vi "CPP_ExponentialDecayFitDevelopment.vi"(4 "MedianFilter(points)":i32=3, 5 "SamplingRate":dbl, 6 "DecayData":dbl[](array[numeric]), 7 "FID ID":string) -> (0 "PlugInValues":string[](array[string]), 1 "smoothedCluster":T2, 2 "GraphClusterArray":T1(array[cluster]), 3 "PlugInTitles":string[](array[string]))   [LabVIEW 2012]
uses:
  <vilib>/measure/mascope.llb/Amplitude and Levels 1 chan.vi
  <vilib>/addons/Time Series Analysis/Series Preprocess.llb/TSA Moving Average (Array).vi
  <vilib>/Analysis/baseanly.llb/Mean (DBL).vi
  <vilib>/Analysis/NI_AALPro.lvlib
  <vilib>/Analysis/NI_AALBase.lvlib
  <vilib>/addons/_Advanced Signal Processing/NI_AdvSigProcTSA.lvlib
  <vilib>/measure/NI_MAPro.lvlib
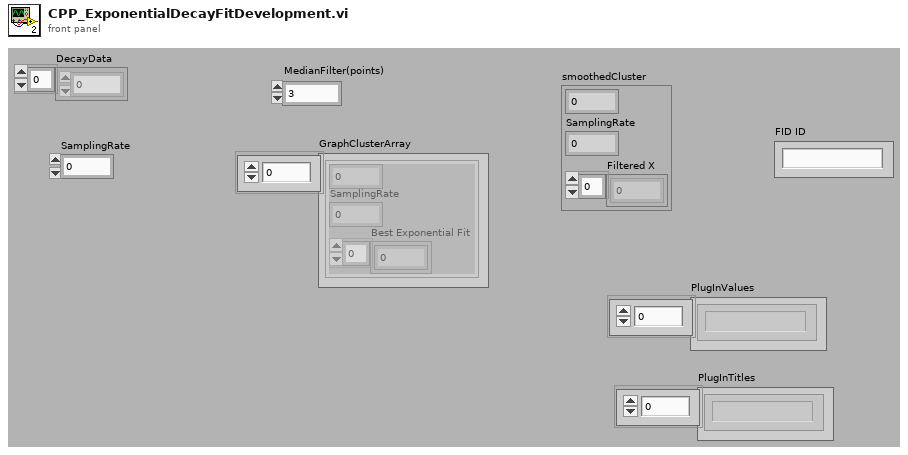
[diagram p1: front panel]
types:
  T1 = cluster{dbl, "SamplingRate":dbl, "Best Exponential Fit":dbl[]}[]
  T2 = cluster{"x*y":dbl, "SamplingRate":dbl, "Filtered X":dbl[]}
  T3 = cluster{dbl, "SamplingRate":dbl, "Best Exponential Fit":dbl[]}
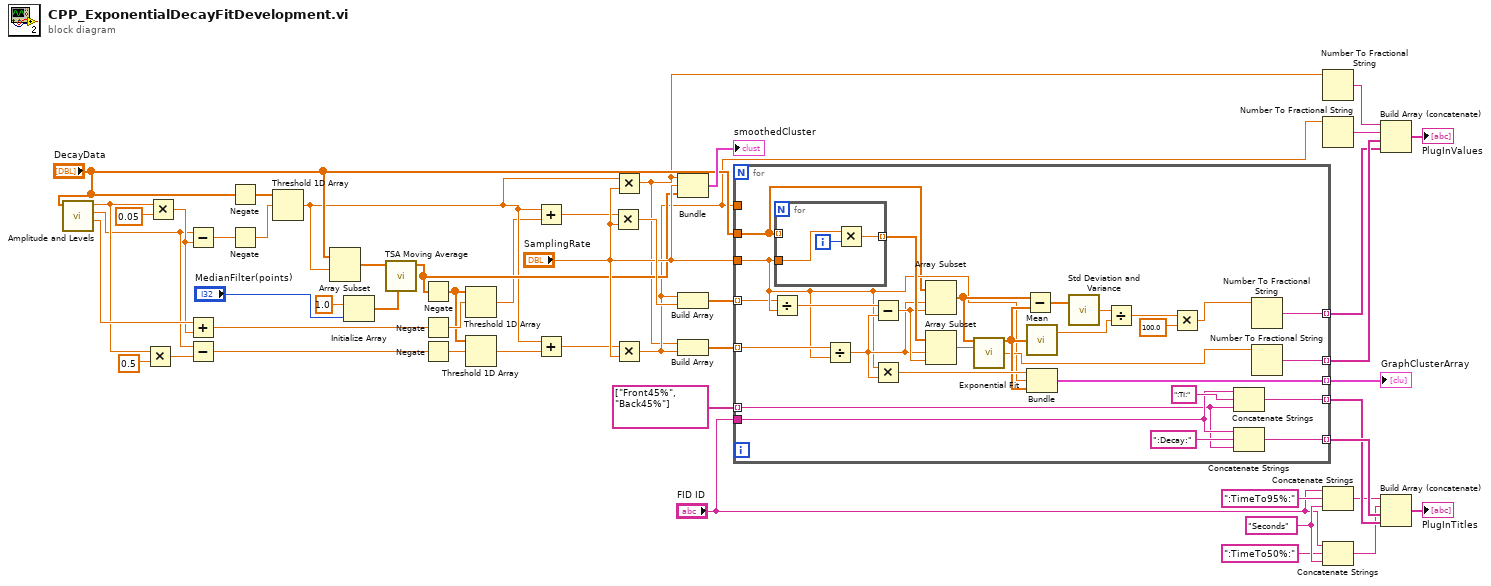
[diagram p0: block diagram]
diagram:
  w11 = "Seconds" ("string")
  n1 = call-poly <vilib>:"Amplitude and Levels.vi"("signal in"="DecayData") -> ("low state level"=w38:dbl, "high state level"=w28:dbl, "amplitude"=w34:dbl)  [unwired: 7 in, 1 out]
  n2 = Multiply(x=w34, y=0.5) -> (x*y=w27:dbl)
  n3 = Multiply(x=w34, y=0.05) -> (x*y=w37:dbl)
  n4 = Subtract(x=w28, y=w37) -> (x-y=w36:dbl)
  n5 = Add(x=w38, y=w37) -> (x+y=w35:dbl)
  n6 = Subtract(x=w28, y=w27) -> (x-y=w26:dbl)
  n7 = Negate(x="DecayData") -> (-x=w25:dbl[])
  n8 = Negate(x=w36) -> (-x=w40:dbl)
  n9 = Threshold 1D Array(2:w40, 3:w25) -> (0:w14:dbl)  [unwired: 1 in]
  n10 = Array Subset(array="DecayData", index=w14) -> (w19:dbl[])  [unwired: 1 in]
  n11 = Initialize Array(1.0 ("element"), "MedianFilter(points)") -> (w21:dbl[])
  n12 = call-poly <vilib>:"TSA Moving Average.vi"("user defined weights"=w21, "Xt"=w19) -> ("Xt out"=w16:dbl[])  [unwired: 8 in, 1 out]
  n13 = Negate(x=w16) -> (-x=w15:dbl[])
  n14 = Negate(x=w35) -> (-x=w39:dbl)
  n15 = Negate(x=w26) -> (-x=w24:dbl)
  n16 = Threshold 1D Array(2:w39, 3:w15) -> (0:w13:dbl)  [unwired: 1 in]
  n17 = Threshold 1D Array(2:w24, 3:w15) -> (0:w18:dbl)  [unwired: 1 in]
  n18 = Add(x=w14, y=w13) -> (x+y=w12:dbl)
  n19 = Add(x=w14, y=w18) -> (x+y=w17:dbl)
  n20 = Multiply(x=w12, y="SamplingRate") -> (x*y=w32:dbl)
  n21 = Multiply(x=w14, y="SamplingRate") -> (x*y=w2:dbl)
  n22 = Multiply(x=w17, y="SamplingRate") -> (x*y=w4:dbl)
  n23 = Bundle(w2, "SamplingRate"="SamplingRate", "Xt out"=w16) -> (→"smoothedCluster":cluster{dbl, "SamplingRate":dbl, "Xt out":dbl[]})  [unwired: 1 out]
  n24 = Build Array(w4, w32) -> (w31:dbl[])
  n25 = Build Array(w2, w4) -> (w30:dbl[])
  n26 = for {
    tunnel: [w73] -> w48 mode=indexing
    tunnel: "DecayData" -> [w53]
    tunnel: w30 -> [w55] mode=indexing
    tunnel: "SamplingRate" -> [w54]
    tunnel: w31 -> [w52] mode=indexing
    tunnel: [w56] -> w46 mode=indexing
    tunnel: [w57] -> w47 mode=indexing
    tunnel: [w60] -> w45 mode=indexing
    tunnel: [w58] -> w44 mode=indexing
    tunnel: w4 -> [_]
    tunnel: "FID ID" -> [w51]
    tunnel: string[] ["Front45%", "Back45%"] -> [w50] mode=indexing
    n27 = Divide(x=w52, y=w54) -> (x/y=w63:dbl)
    n28 = for {
      tunnel: w53 -> [_] mode=indexing
      tunnel: w54 -> [w79]
      tunnel: [w78] -> w77 mode=indexing
      i -> [w80]
      n29 = Multiply(x=w79, y=w80) -> (x*y=w78:dbl)
    }
    n30 = Divide(x=w55, y=w54) -> (x/y=w64:dbl)
    n31 = Subtract(x=w63, y=w64) -> (x-y=w76:dbl)
    n32 = Multiply(x=w54, y=w64) -> (x*y=w74:dbl)
    n33 = Array Subset(array=w53, index=w64, length=w76) -> (w72:dbl[])
    n34 = Array Subset(array=w77, index=w64, length=w76) -> (w75:dbl[])
    n35 = call <vilib>:"Exponential Fit.vi"("Y"=w72, "X"=w75) -> ("Best Exponential Fit"=w70:dbl[], "damping"=w61:dbl)  [unwired: 8 in, 4 out]
    n36 = Subtract(x=w72, y=w70) -> (x-y=w71:dbl[])
    n37 = call-poly <vilib>:"Mean.vi"("X"=w70) -> ("mean"=w68:dbl)  [unwired: 1 out]
    n38 = Bundle(w74, "SamplingRate"=w54, "Best Exponential Fit"=w70) -> (w73:T3)  [unwired: 1 out]
    n39 = call <vilib>:"Std Deviation and Variance.vi"("X"=w71) -> ("standard deviation"=w69:dbl)  [unwired: 1 in, 2 out]
    n40 = Divide(x=w69, y=w68) -> (x/y=w67:dbl)
    n41 = Multiply(x=w67, y=100.0) -> (x*y=w59:dbl)
    n42 = Concatenate Strings(w51, ":TI:" ("string"), w50) -> (w56:string)
    n43 = Concatenate Strings(w51, ":Decay:" ("string"), w50) -> (w57:string)
    n44 = Number To Fractional String(number=w59) -> (F-format string=w58:string)  [unwired: 3 in]
    n45 = Number To Fractional String(number=w61) -> (F-format string=w60:string)  [unwired: 3 in]
  }
  "GraphClusterArray" <- w48
  n46 = Number To Fractional String(number=w2) -> (F-format string=w1:string)  [unwired: 3 in]
  n47 = Number To Fractional String(number=w4) -> (F-format string=w3:string)  [unwired: 3 in]
  n48 = Concatenate Strings("FID ID", ":TimeTo95%:" ("string"), w11) -> (w5:string)
  n49 = Concatenate Strings("FID ID", ":TimeTo50%:" ("string"), w11) -> (w6:string)
  n50 = Build Array (concatenate)(w1, w3, w45, w44) -> (→"PlugInValues":string[])
  n51 = Build Array (concatenate)(w5, w6, w47, w46) -> (→"PlugInTitles":string[])
